vi "BartlomiejLechman_prac9_3.vi"   [LabVIEW 2019]
types:
  T1 = enum16{"open", "replace", "create", "open or create", "replace or create", "replace or create with confirmation"}
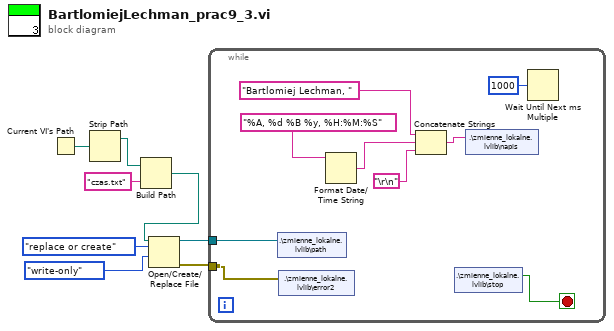
[diagram p0: block diagram]
diagram:
  n1 = Current VI's Path() -> (path=w8:path)
  n2 = Strip Path(path=w8) -> (stripped path=w7:path)  [unwired: 1 out]
  n3 = Build Path(base path=w7, name or relative path="czas.txt") -> (appended path=w3:path)
  n4 = Open/Create/Replace File(file path (use dialog)=w3, operation (0:open)=T1."replace or create", access (0:read/write)=enum16{"read/write", "read-only", "write-only"}."write-only") -> (refnum out=w1:refnum<file>, error out=w2:errorcluster)  [unwired: 3 in, 1 out]
  n5 = while {
    tunnel: w2 -> [w9]
    tunnel: w1 -> [w10]
    stop <- w17 stop-if-true
    n6 = shared-variable ".\\zmienne_lokalne.lvlib\\path"(w10) -> ()  [unwired: 1 in, 1 out]
    n7 = shared-variable ".\\zmienne_lokalne.lvlib\\error2"(w9) -> ()  [unwired: 1 in, 1 out]
    n8 = Format Date/Time String(time format string (%c)="%A, %d %B %y, %H:%M:%S") -> (date/time string=w13:string)  [unwired: 2 in]
    n9 = Concatenate Strings("Bartlomiej Lechman, " ("string"), w13, "\r\n") -> (w11:string)
    n10 = shared-variable ".\\zmienne_lokalne.lvlib\\stop"() -> (w17:bool)  [unwired: 1 in, 1 out]
    n11 = shared-variable ".\\zmienne_lokalne.lvlib\\napis"(w11) -> ()  [unwired: 1 in, 1 out]
    n12 = Wait Until Next ms Multiple(millisecond multiple=u32 1000) -> ()  [unwired: 1 out]
  }
